vi "System A Temp Curve.vi"(2 "Sorb Goal Temp":dbl min=0.0 max=45.0 step=1e-05, 3 "He3 Goal Temp":dbl min=0.0 max=1.4 step=1e-05) -> (0 "Corresponding He3 Temp":dbl, 1 "Corresponding Sorb Temp":dbl)   [LabVIEW 2024]
uses:
  <vilib>/Utility/file.llb/Read Delimited Spreadsheet (DBL).vi
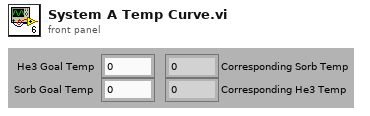
[diagram p1: front panel]
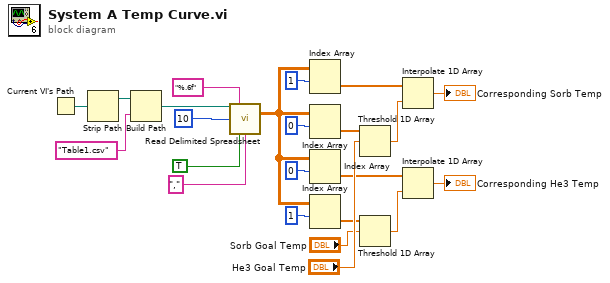
[diagram p0: block diagram]
diagram:
  n1 = Current VI's Path() -> (path=w16:path)
  n2 = Strip Path(path=w16) -> (stripped path=w15:path)  [unwired: 1 out]
  n3 = Build Path(base path=w15, name or relative path="Table1.csv") -> (appended path=w2:path)
  n4 = call-poly <vilib>:"Read Delimited Spreadsheet.vi"("file path (dialog if empty)"=w2, "format (%.3f)"="%.6f", "start of read offset (chars.:0)"=10, "transpose? (F)"=TRUE ("transpose (no:F)"), "delimiter (\\t)"="," ("delimiter (\\t)")) -> ("all rows"=w1:dbl[][])  [unwired: 5 in, 5 out]
  n5 = Index Array(array=w1, index (row)=1) -> (element=w19:dbl[])  [unwired: 1 in]
  n6 = Index Array(array=w1, index (row)=0) -> (element=w22:dbl[])  [unwired: 1 in]
  n7 = Index Array(array=w1, index (row)=0) -> (element=w10:dbl[])  [unwired: 1 in]
  n8 = Index Array(array=w1, index (row)=1) -> (element=w12:dbl[])  [unwired: 1 in]
  n9 = Threshold 1D Array(2:"He3 Goal Temp", 3:w22) -> (0:w18:dbl)  [unwired: 1 in]
  n10 = Threshold 1D Array(2:"Sorb Goal Temp", 3:w12) -> (0:w7:dbl)  [unwired: 1 in]
  n11 = Interpolate 1D Array(1:w18, 2:w19) -> (0:→"Corresponding Sorb Temp":dbl)
  n12 = Interpolate 1D Array(1:w7, 2:w10) -> (0:→"Corresponding He3 Temp":dbl)
